vi "rest_get_devices.vi"(8 "error in":errorcluster) -> (0 "error out":errorcluster, 2 "DeviceArray":string[](array[string]))   [LabVIEW 2024]
uses:
  <vilib>/addons/_JKI.lib/REST Client/classes/REST Client/REST Client.lvclass
panel:
  in  "Base URL":string="http://localhost:5001/"
  out "Menu Ring":u16(ring) items=["esp32-t222", "esp32-test", "esp32-t333", "esp32-t101"]
  out "Devices":cluster{"device_id":string}[](array[cluster])
  out "Response body":string
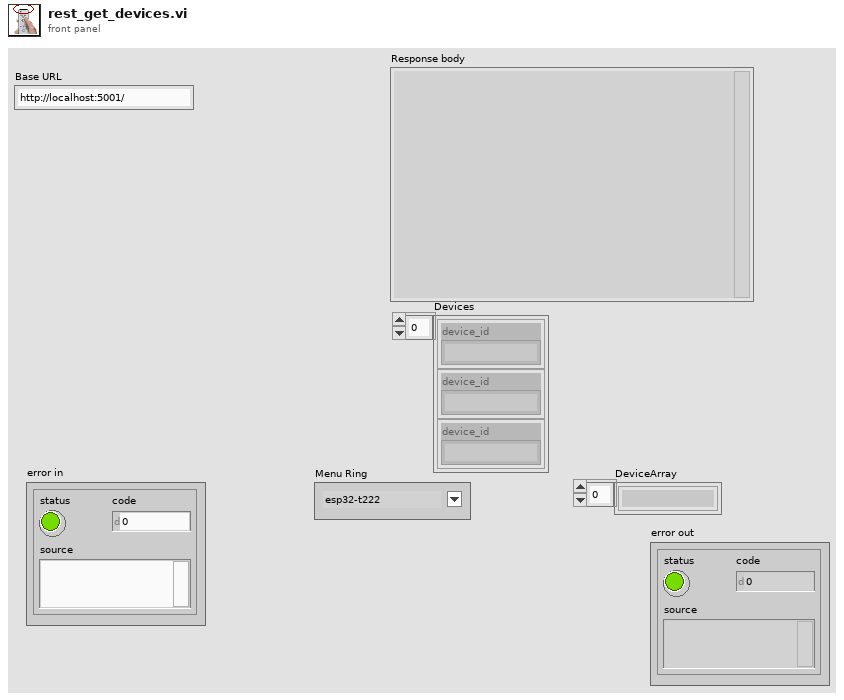
[diagram p1: front panel]
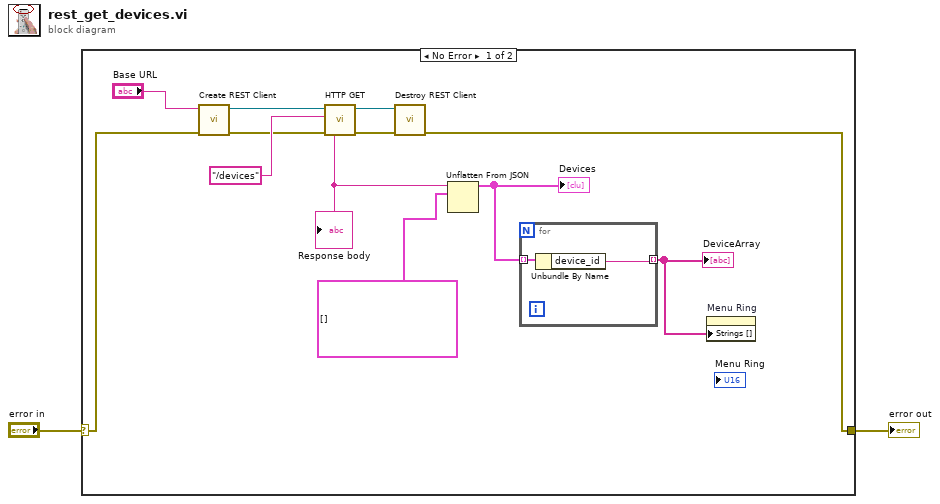
[diagram p0: block diagram]
diagram:
  n1 = case shown="No Error" "error in" {
    selector: "error in" -> [w6 w17]
    tunnel: [w3 w17] -> w1
    frame No Error {
      n2 = call <vilib>:"Create REST Client.vi"("error in (no error)"=w6, "Base URL"="Base URL") -> ("error out"=w5:errorcluster, "REST Client out"=w14:refnum<class "REST Client.lvclass">)  [unwired: 8 in]
      n3 = call-dynamic "HTTP GET.vi"("error in (no error)"=w5, "Path"="/devices", "REST Client in"=w14) -> ("error out"=w4:errorcluster, "Response body"=w10:string, "REST Client out"=w13:refnum<class "REST Client.lvclass">)  [unwired: 3 in, 3 out]
      "Response body" <- w10
      n4 = call-dynamic "Destroy REST Client.vi"("error in (no error)"=w4, "REST Client in"=w13) -> ("error out"=w3:errorcluster)  [unwired: 9 in]
      n5 = Unflatten From JSON(JSON string=w10, type and defaults=cluster{"device_id":string}[] []) -> (value=w8:cluster{"device_id":string}[])  [unwired: 5 in, 1 out]
      "Devices" <- w8
      n6 = for {
        tunnel: w8 -> [w16] mode=indexing
        tunnel: [w15] -> w7 mode=indexing
        n7 = Unbundle By Name(w16) -> ("device_id"=w15:string)
      }
      "DeviceArray" <- w7
      n8 = property on="Menu Ring" class="Ring (strict)"("Strings []"=w7) -> ()  [unwired: 2 in, 2 out]
    }
    frame Error {
    }
  }
  "error out" <- w1
